vi "ControllerTest.vi"() -> ()   [LabVIEW 2013]
uses:
  <vilib>/Utility/inputDevices.llb/joystickAcquire.vi
  ManualControlGlobal.vi
panel:
  out "TTspeed":dbl
  in  "Stop Button":bool
  out "direction info":T1
  out "button info":T2
  out "axis info":T3
  in  "device index":i32
  out "joystick info":T4(array[cluster])
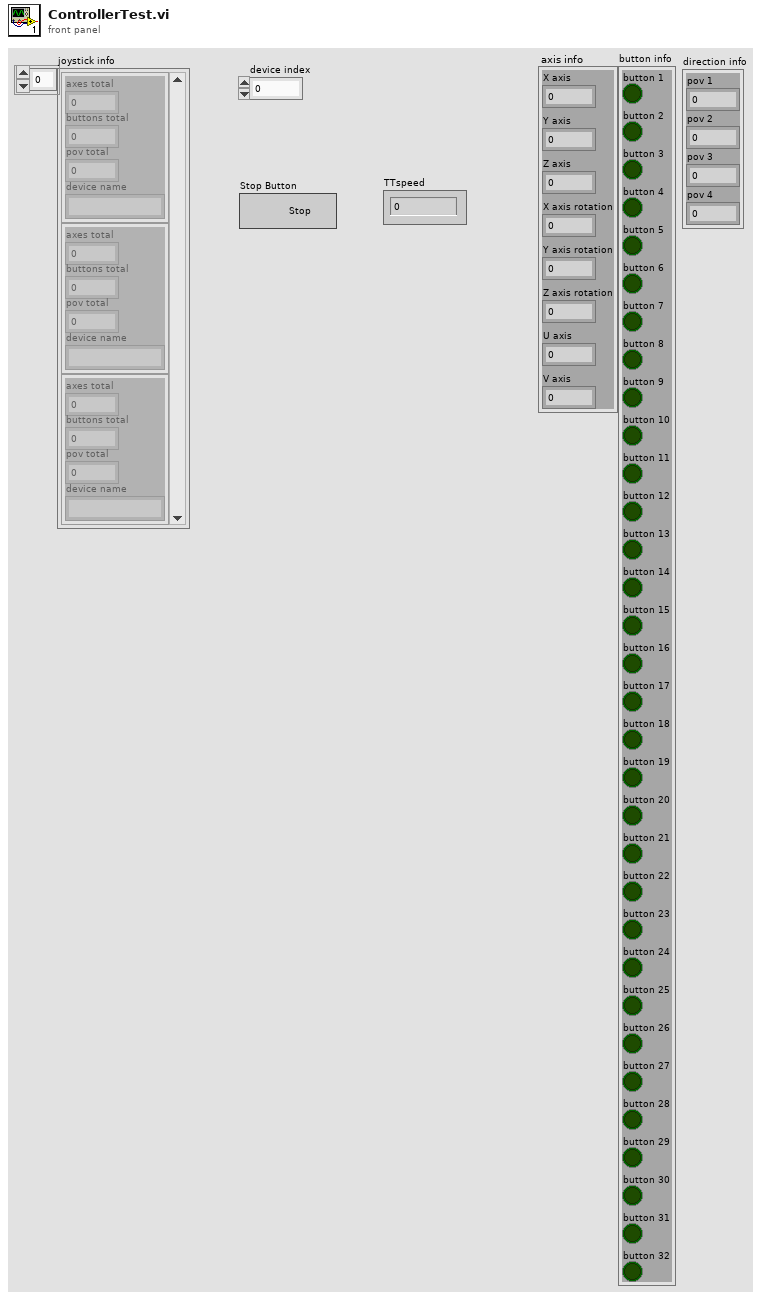
[diagram p1: front panel]
types:
  T1 = cluster{"pov 1":i32, "pov 2":i32, "pov 3":i32, "pov 4":i32}
  T2 = cluster{"button 1":bool, "button 2":bool, "button 3":bool, "button 4":bool, "button 5":bool, "button 6":bool, "button 7":bool, "button 8":bool, "button 9":bool, "button 10":bool, "button 11":bool, "button 12":bool, "button 13":bool, "button 14":bool, "button 15":bool, "button 16":bool, "button 17":bool, "button 18":bool, "button 19":bool, "button 20":bool, "button 21":bool, "button 22":bool, "button 23":bool, "button 24":bool, "button 25":bool, "button 26":bool, "button 27":bool, "button 28":bool, "button 29":bool, "button 30":bool, "button 31":bool, "button 32":bool}
  T3 = cluster{"X axis":i32, "Y axis":i32, "Z axis":i32, "X axis rotation":i32, "Y axis rotation":i32, "Z axis rotation":i32, "U axis":i32, "V axis":i32}
  T4 = cluster{"axes total":u32, "buttons total":u32, "pov total":u32, "device name":string}[]
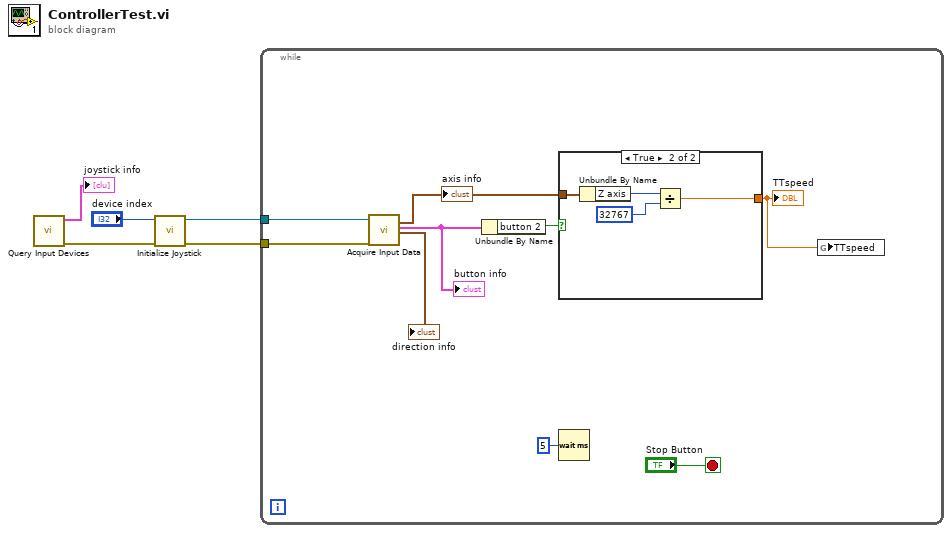
[diagram p0: block diagram]
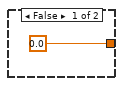
[diagram p2: hidden frame]
diagram:
  n1 = call <vilib>:"Query Input Devices.vi"() -> ("error out"=w5:errorcluster, "joystick info"=→"joystick info":T4)  [unwired: 1 in, 9 out]
  n2 = call <vilib>:"Initialize Joystick.vi"("error in (no error)"=w5, "device index"="device index") -> ("error out"=w4:errorcluster, "device ID"=w1:refnum<k1>)  [unwired: 8 out]
  n3 = while {
    tunnel: w4 -> [w14]
    tunnel: w1 -> [w13]
    stop <- "Stop Button" stop-if-true
    n4 = call-poly <vilib>:"Acquire Input Data.vi"("device ID"=w13, "error in (no error)"=w14) -> ("axis info"=w9:T3, "button info"=w8:T2, "direction info"=→"direction info":T1)  [unwired: 15 out]
    "axis info" <- w9
    "button info" <- w8
    n5 = Unbundle By Name(w8) -> ("button 2"=w7:bool)
    n6 = case shown="True" w7 {
      tunnel: w9 -> [_ w19]
      tunnel: [0.0 w16] -> w6
      frame False {
      }
      frame True {
        n7 = Unbundle By Name(w19) -> ("Z axis"=w18:i32)
        n8 = Divide(x=w18, y=32767) -> (x/y=w16:dbl)
      }
    }
    "TTspeed" <- w6
    n9 = Wait (ms)(milliseconds to wait=u32 5) -> ()  [unwired: 1 out]
    n10 = global write "ManualControlGlobal.vi" "TTspeed"(w6) -> ()
  }
